vi "App_Configuration(FGV).vi"(6 "Config Method(Get)":T1, 8 "error in":errorcluster, 11 "Configuration In":T2) -> (0 "error out":errorcluster, 3 "Configuration Out":T2)   [LabVIEW 2015, in "Application 2.lvlib"]
uses:
  Application 2.lvlib
  Data Def/App_Configuration.ctl
  Data Def/App_Config Method.ctl
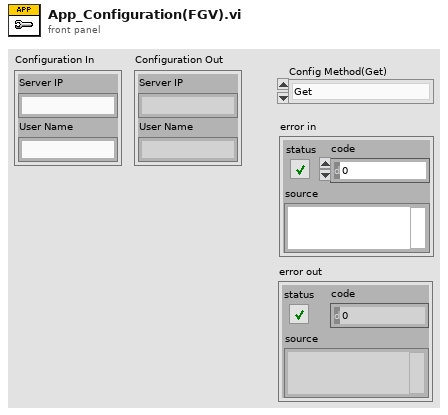
[diagram p1: front panel]
types:
  T1 = typedef "Application 2.lvlib/App_Config Method.ctl" = enum16{"Get", "Put", "Load", "Save"}
  T2 = typedef "Application 2.lvlib/App_Configuration.ctl" = cluster{"Server IP":string, "User Name":string}
  T3 = enum16{"open", "replace", "create", "open or create", "replace or create", "replace or create with confirmation"}
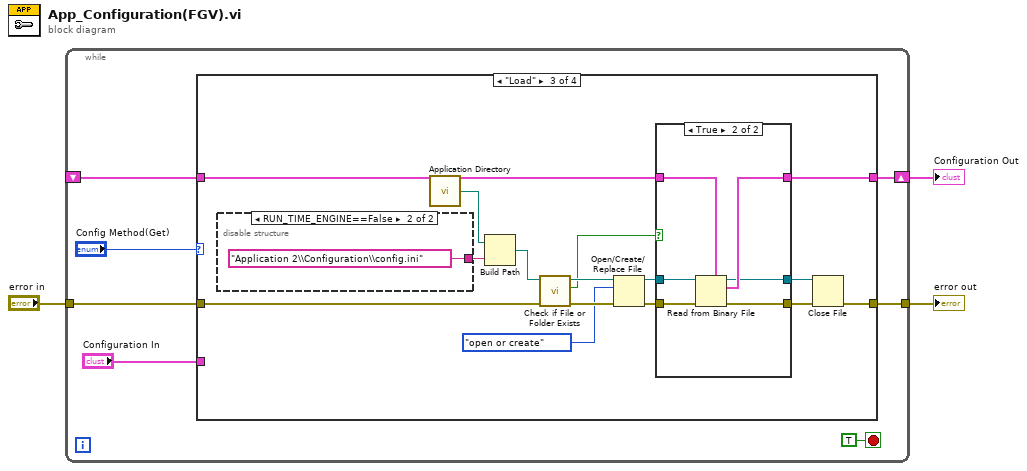
[diagram p0: block diagram]
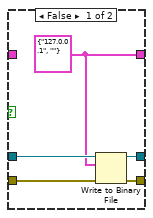
[diagram p4: hidden frame]
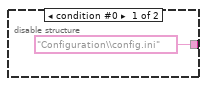
[diagram p5: hidden frame]
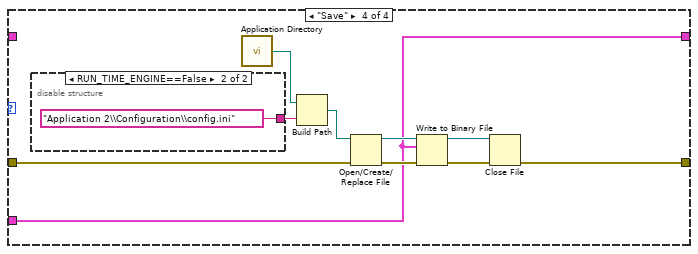
[diagram p6: hidden frame]
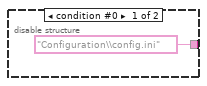
[diagram p7: hidden frame]
diagram:
  n1 = while {
    tunnel: "error in" -> [w7]
    shift-right: [w6] -> w1
    shift-left: _ -> [w5]
    tunnel: [w4] -> w2
    stop <- TRUE stop-if-true
    n2 = case shown="\"Load\"" "Config Method(Get)" {
      tunnel: "Configuration In" -> [_ w14 _ w43]
      tunnel: w7 -> [w11 w13 w27 w50]
      tunnel: [w12 w14 w19 w43] -> w6
      tunnel: w5 -> [w12 _ w18 _]
      tunnel: [w11 w13 w15 w44] -> w4
      frame "Get", Default {
      }
      frame "Put" {
      }
      frame "Load" {
        n3 = disable-structure shown="RUN_TIME_ENGINE==False" {
          disable-tunnel: ["Configuration\\config.ini" ("name or relative path") "Application 2\\Configuration\\config.ini" ("name or relative path")] -> w29
          frame condition #0 {
          }
          frame condition #1 (active) {
          }
        }
        n4 = call <vilib>:"Application Directory.vi"() -> ("Application Directory"=w28:path)
        n5 = Build Path(base path=w28, name or relative path=w29) -> (appended path=w26:path)
        n6 = call <vilib>:"Check if File or Folder Exists.vi"("error in (no error)"=w27, "path"=w26) -> ("error out"=w25:errorcluster, "file or folder exists?"=w22:bool, "dup path"=w24:path)  [unwired: 7 in]
        n7 = Open/Create/Replace File(file path (use dialog)=w24, error in=w25, operation (0:open)=T3."open or create") -> (refnum out=w21:refnum<file>, error out=w20:errorcluster)  [unwired: 3 in, 1 out]
        n8 = case shown="True" w22 {
          tunnel: w21 -> [w31 w39]
          tunnel: w20 -> [w34 w40]
          tunnel: [w30 w38] -> w19
          tunnel: w18 -> [_ w37]
          tunnel: [w33 w36] -> w17
          tunnel: [w32 w35] -> w16
          frame False {
            w30 = T2 {"Server IP"="127.0.0.1", "User Name"=""} ("Configuration In")
            n9 = Write to Binary File(file (use dialog)=w31, data=w30, error in=w34) -> (refnum out=w32:refnum<file>, error out=w33:errorcluster)  [unwired: 3 in, 1 out]
          }
          frame True {
            n10 = Read from Binary File(5:w37, 8:w40, 11:w39) -> (0:w36:errorcluster, 2:w38:T2, 3:w35:refnum<file>)  [unwired: 3 in, 1 out]
          }
        }
        n11 = Close File(refnum=w16, error in=w17) -> (error out=w15:errorcluster)  [unwired: 1 out]
      }
      frame "Save" {
        n12 = disable-structure shown="RUN_TIME_ENGINE==False" {
          disable-tunnel: ["Configuration\\config.ini" ("name or relative path") "Application 2\\Configuration\\config.ini" ("name or relative path")] -> w52
          frame condition #0 {
          }
          frame condition #1 (active) {
          }
        }
        n13 = call <vilib>:"Application Directory.vi"() -> ("Application Directory"=w51:path)
        n14 = Build Path(base path=w51, name or relative path=w52) -> (appended path=w49:path)
        n15 = Open/Create/Replace File(file path (use dialog)=w49, error in=w50) -> (refnum out=w47:refnum<file>, error out=w48:errorcluster)  [unwired: 4 in, 1 out]
        n16 = Write to Binary File(file (use dialog)=w47, data=w43, error in=w48) -> (refnum out=w45:refnum<file>, error out=w46:errorcluster)  [unwired: 3 in, 1 out]
        n17 = Close File(refnum=w45, error in=w46) -> (error out=w44:errorcluster)  [unwired: 1 out]
      }
    }
  }
  "Configuration Out" <- w1
  "error out" <- w2
